vi "Erase (index).vi"(8 "error in (no error)":errorcluster, 10 "Index":i32, 11 "Parameter to Hardware Map in":refnum<class "Parameter to Hardware Map.lvclass">) -> (0 "error out":errorcluster, 2 "Deleted Pair":T1, 3 "Parameter to Hardware Map out":refnum<class "Parameter to Hardware Map.lvclass">)   [LabVIEW 2020, in "Parameter to Hardware Map.lvclass"]
doc: "Removes the element from the map specified by the given index."
uses:
  Parameter to Hardware Map.lvclass
  Controller/Generic Plugin.lvclass
  Pair.ctl
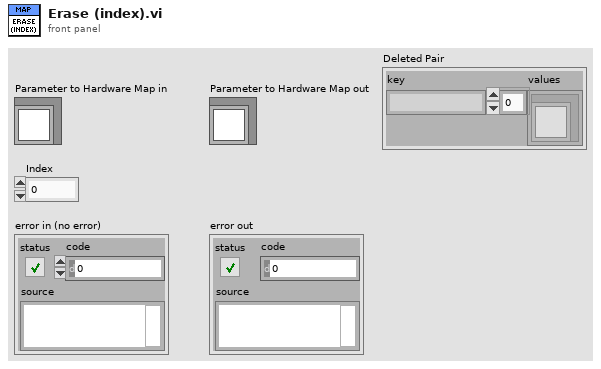
[diagram p1: front panel]
types:
  T1 = typedef "Parameter to Hardware Map.lvclass/Pair.ctl" = cluster{"key":string, "values":refnum<class "Generic Plugin.lvclass">[]}
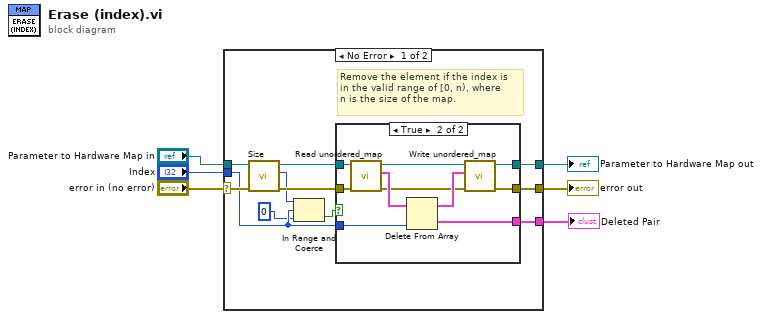
[diagram p0: block diagram]
diagram:
  n1 = case shown="No Error" "error in (no error)" {
    selector: "error in (no error)" -> [w13 w30]
    tunnel: [w17 w30] -> w6
    tunnel: [w16 w31] -> w5
    tunnel: "Index" -> [w9 _]
    tunnel: "Parameter to Hardware Map in" -> [w15 w31]
    tunnel: [w7 _] -> w1
    frame No Error {
      # "Remove the element if the index is\nin the valid range of [0, n), where \nn is the size of the map."
      n2 = call "Size.vi"("error in (no error)"=w13, "Parameter to Hardware Map in"=w15) -> ("error out"=w12:errorcluster, "Size"=w10:i32, "Parameter to Hardware Map out"=w14:refnum<class "Parameter to Hardware Map.lvclass">)  [unwired: 7 in]
      n3 = In Range and Coerce(upper limit=w10, x=w9, lower limit=0) -> (In Range?=w11:bool)  [unwired: 1 out]
      n4 = case shown="True" w11 {
        tunnel: [w18 w29] -> w17
        tunnel: [w19 w28] -> w16
        tunnel: w9 -> [_ w27]
        tunnel: w14 -> [w19 w22]
        tunnel: w12 -> [w18 w21]
        tunnel: [_ w20] -> w7
        frame False {
        }
        frame True {
          n5 = call "Read unordered_map.vi"("error in (no error)"=w21, "Parameter to Hardware Map in"=w22) -> ("error out"=w23:errorcluster, "unordered_map"=w24:T1[], "Parameter to Hardware Map out"=w25:refnum<class "Parameter to Hardware Map.lvclass">)  [unwired: 7 in]
          n6 = Delete From Array(array=w24, index=w27) -> (deleted portion=w20:T1, array with subset deleted=w26:T1[])  [unwired: 1 in]
          n7 = call "Write unordered_map.vi"("error in (no error)"=w23, "unordered_map"=w26, "Parameter to Hardware Map in"=w25) -> ("error out"=w29:errorcluster, "Parameter to Hardware Map out"=w28:refnum<class "Parameter to Hardware Map.lvclass">)  [unwired: 7 in]
        }
      }
    }
    frame Error {
    }
  }
  "error out" <- w6
  "Parameter to Hardware Map out" <- w5
  "Deleted Pair" <- w1
